vi "Read Data.vi"(7 "UART":refnum<class "UART.lvclass">, 8 "error in (no error)":errorcluster, 9 "Len (LineTerm)":u8, 11 "Session In":refnum<class "Session.lvclass">) -> (0 "error out":errorcluster, 1 "Data":string, 3 "Session Out":refnum<class "Session.lvclass">)   [LabVIEW 2020, in "CTI.lvlib" / "UART.lvclass"]
uses:
  UART.lvclass
  UART.lvclass/UART.ctl
  Session/Session.lvclass
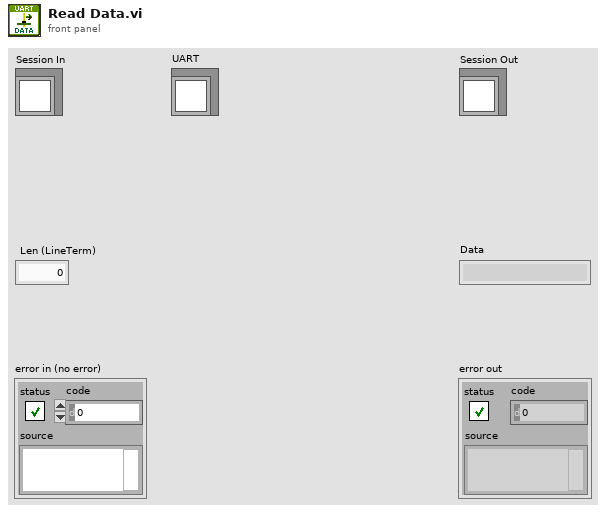
[diagram p1: front panel]
types:
  T1 = typedef "CTI.lvlib/UART Number.ctl" = i8
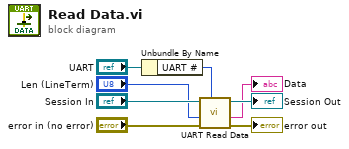
[diagram p0: block diagram]
diagram:
  n1 = Unbundle By Name("UART") -> ("UART #"=w3:T1)
  n2 = call "UART Read Data.vi"("UART #"=w3, "error in (no error)"="error in (no error)", "Len (LineTerm)"="Len (LineTerm)", "Session in"="Session In") -> ("error out"=→"error out":errorcluster, "Data"=→"Data":string, "Session out"=→"Session Out":refnum<class "Session.lvclass">)  [unwired: 5 in]
